vi "Write Tempo de espera.vi"(8 "error in (no error)":errorcluster, 10 "Tempo de espera":u16, 11 "CCDCamera in":refnum<class "CCDCamera.lvclass">) -> (0 "error out":errorcluster, 3 "CCDCamera out":refnum<class "CCDCamera.lvclass">)   [LabVIEW 2018, in "CCDCamera.lvclass"]
uses:
  CCDCamera.lvclass
  CCDCamera.lvclass/CCDCamera.ctl
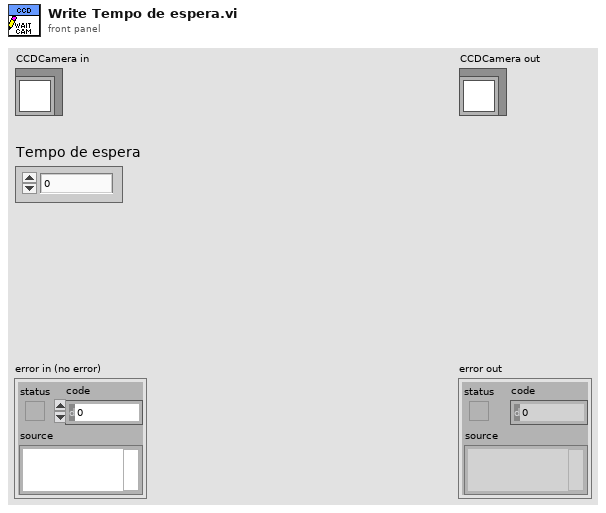
[diagram p1: front panel]
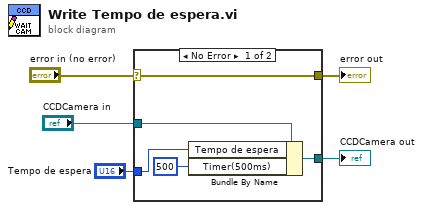
[diagram p0: block diagram]
diagram:
  n1 = case shown="No Error" "error in (no error)" {
    selector: "error in (no error)" -> [w10 w11]
    tunnel: [w10 w11] -> w4
    tunnel: [w8 w12] -> w2
    tunnel: "CCDCamera in" -> [w9 w12]
    tunnel: "Tempo de espera" -> [w7 _]
    frame No Error {
      n2 = Bundle By Name(cluster=w9, "Tempo de espera"=w7, "Timer(500ms)"=u16 500) -> (w8:refnum<class "CCDCamera.lvclass">)
    }
    frame Error {
    }
  }
  "error out" <- w4
  "CCDCamera out" <- w2
